vi "系统配置.vi"() -> (3 "线别配置 2":T2={"线别名称"="A157", "LOT NO"="Z-TEST", "机器名"="1", "作业员ID"="A157"})   [LabVIEW 2014]
uses:
  Button.ctl
panel:
  out "线别[]":T1(array[cluster])
  out "作业员IDout":string="A157"
  out "dup path":path caption="路径副本"
  in  "线别设置 2":T3={"LOT NO"="A157", "机器名"="Z-TEST", "QTY"="1", "ACTIVITY"="", "RESOURCE"="A-6-Z-TEST", "NC_CODE"="Z-TEST_FAIL", "IP"="10.9.30.175", "PORT"="50100", "URL"="/manufacturing/IntegrationServlet?InterType=XML&message="}
  out "MES 配置 2":T4={"线别名称"="A157", "LOT NO"="Z-TEST", "机器名"="1"}
  in  "线别配置":T2={"线别名称"="A157", "LOT NO"="Z-TEST", "机器名"="1", "作业员ID"="A157"}
  in  "delete":T5
  in  "input":T5
  in  "新建":T5
  in  "Exit":T5
  in  "所有线别":i32(listbox)
  in  "线别名称":string
  # "用户配置"
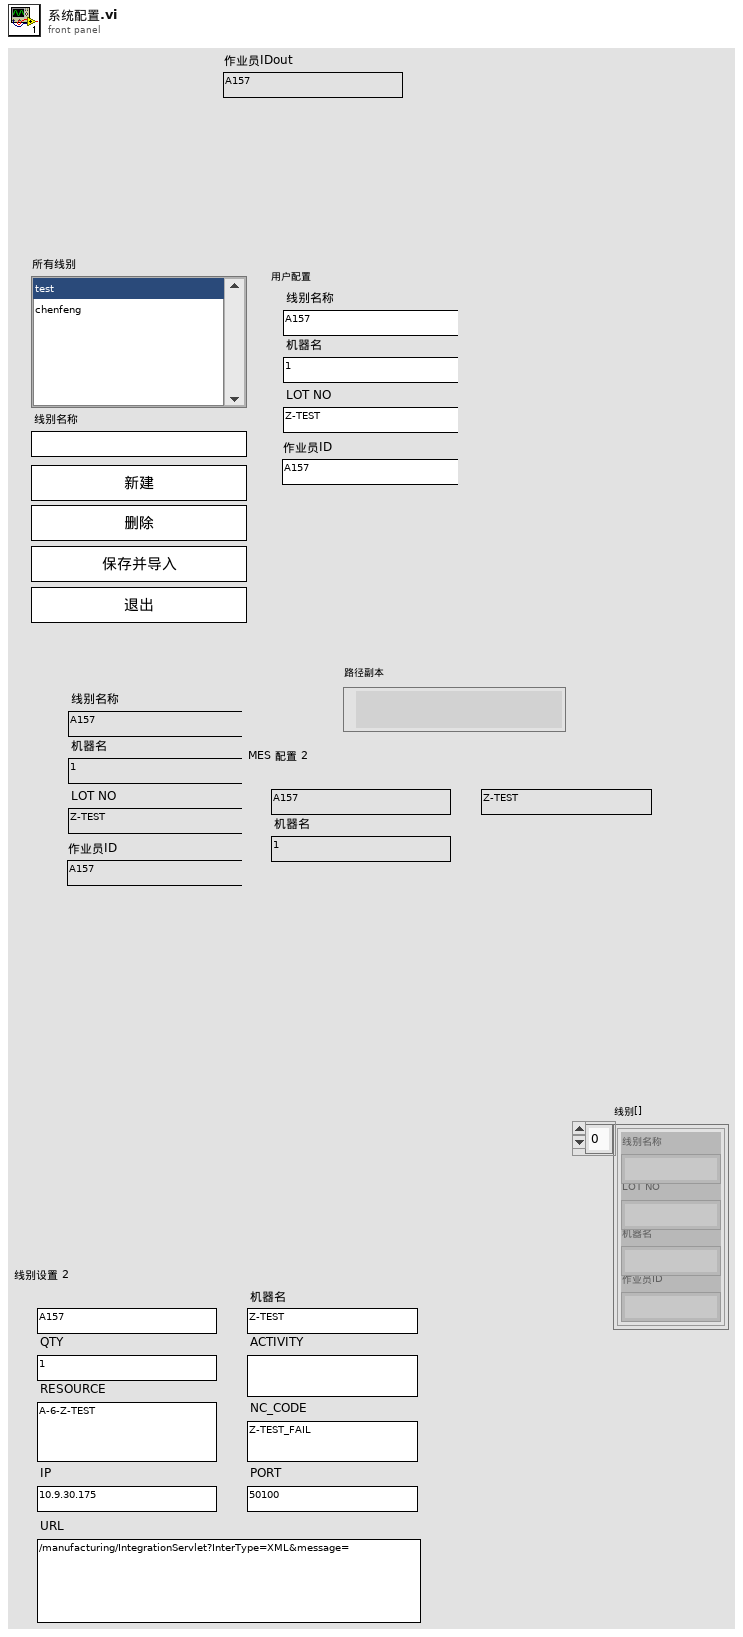
[diagram p1: front panel]
types:
  T1 = cluster{"线别名称":string, "LOT NO":string, "机器名":string, "作业员ID":string}[]
  T2 = cluster{"线别名称":string, "LOT NO":string, "机器名":string, "作业员ID":string}
  T3 = cluster{"LOT NO":string, "机器名":string, "QTY":string, "ACTIVITY":string, "RESOURCE":string, "NC_CODE":string, "IP":string, "PORT":string, "URL":string}
  T4 = cluster{"线别名称":string, "LOT NO":string, "机器名":string}
  T5 = typedef "Button.ctl" = bool
  T6 = cluster{"名称":string, "MES 配置":cluster{"SITE":string, "OPERATION":string, "QTY":string, "ACTIVITY":string, "RESOURCE":string, "NC_CODE":string, "IP":string, "PORT":string, "URL":string}}
  T7 = cluster{"名称":string, "电机位置":cluster{"左工位工作位置":cluster{"Axis":i16, "Distance":i32, "StrVel":i32, "MaxVel":i32}, "左工位抬起开关位置":cluster{"Axis":i16, "Distance":i32, "StrVel":i32, "MaxVel":i32}, "左工位按下开关位置":cluster{"Axis":i16, "Distance":i32, "StrVel":i32, "MaxVel":i32}, "右工位工作位置":cluster{"Axis":i16, "Distance":i32, "StrVel":i32, "MaxVel":i32}, "右工位抬起开关位置":cluster{"Axis":i16, "Distance":i32, "StrVel":i32, "MaxVel":i32}, "右工位按下开关位置":cluster{"Axis":i16, "Distance":i32, "StrVel":i32, "MaxVel":i32}}}
  T8 = cluster{"名称":string, "判定条件":cluster{"A1-A2电阻":cluster{"上限":dbl, "下限":dbl, "单位":string}, "A3-A4电阻":cluster{"上限":dbl, "下限":dbl, "单位":string}, "A4-A5电阻":cluster{"上限":dbl, "下限":dbl, "单位":string}, "A5-A6电阻":cluster{"上限":dbl, "下限":dbl, "单位":string}, "A1-A3电阻":cluster{"上限":dbl, "下限":dbl, "单位":string}, "A2-A6电阻":cluster{"上限":dbl, "下限":dbl, "单位":string}, "A1导地A3-A5电压":cluster{"上限":dbl, "下限":dbl, "单位":string}, "A2导地A6-A5电压":cluster{"上限":dbl, "下限":dbl, "单位":string}, "抬起开关A3-A5电压":cluster{"上限":dbl, "下限":dbl, "单位":string}, "按下开关A6-A5电压":cluster{"上限":dbl, "下限":dbl, "单位":string}, "背光电流":cluster{"上限":dbl, "下限":dbl, "单位":string}, "A1导地A6-A5电压":cluster{"上限":dbl, "下限":dbl, "单位":string}, "A2导地A3-A5电压":cluster{"上限":dbl, "下限":dbl, "单位":string}}}
  T9 = enum16{"open", "replace", "create", "open or create", "replace or create", "replace or create with confirmation"}
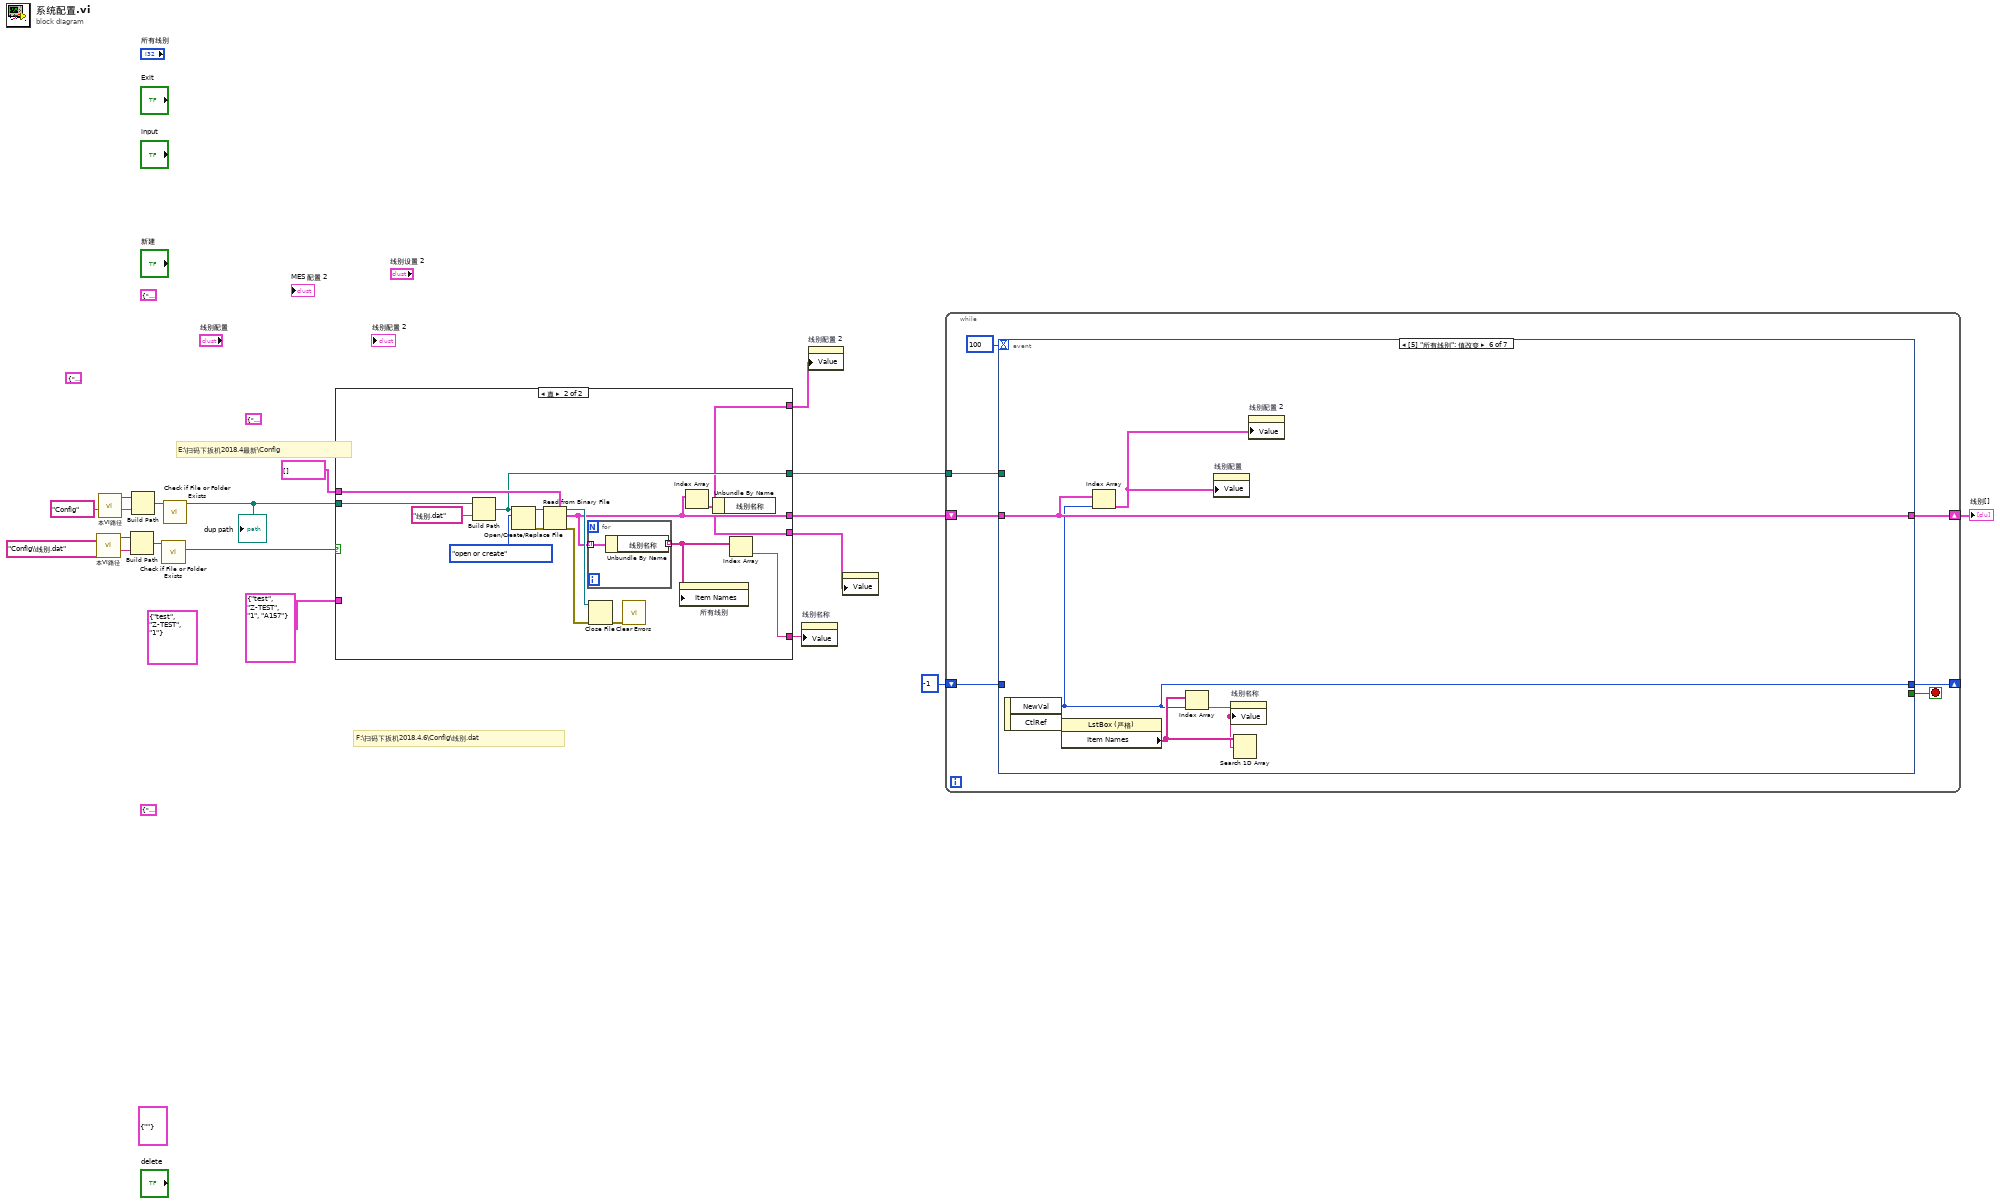
[diagram p0: block diagram]
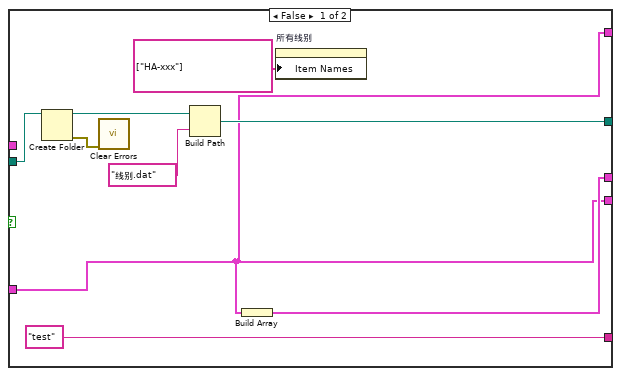
[diagram p2: hidden frame]
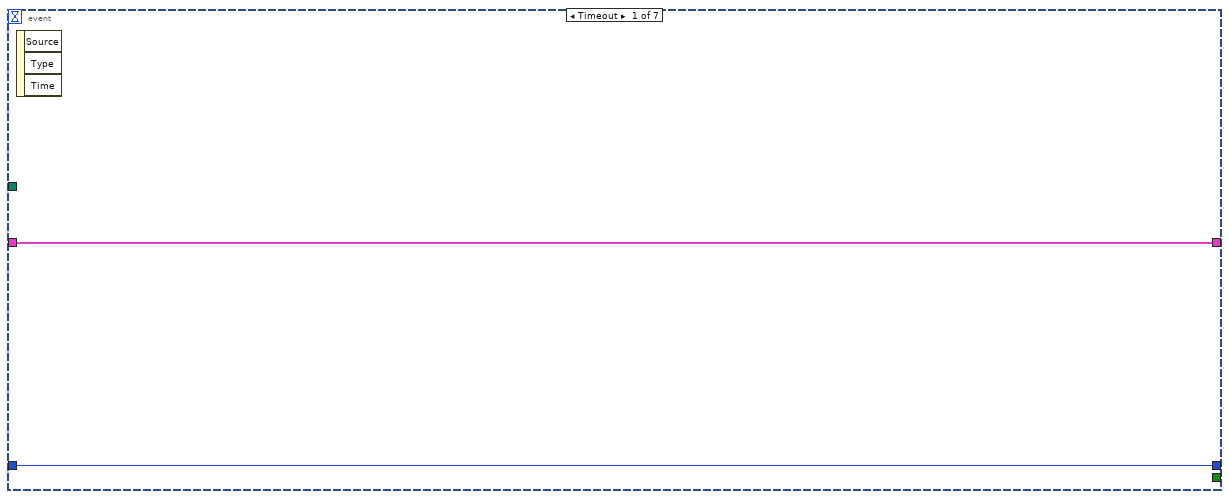
[diagram p3: hidden frame]
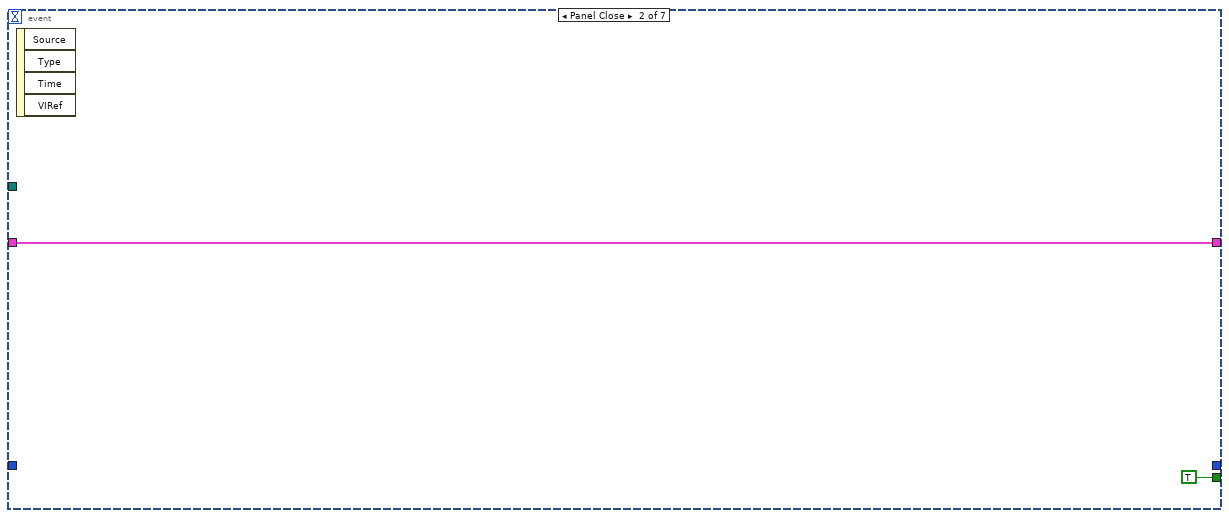
[diagram p4: hidden frame]
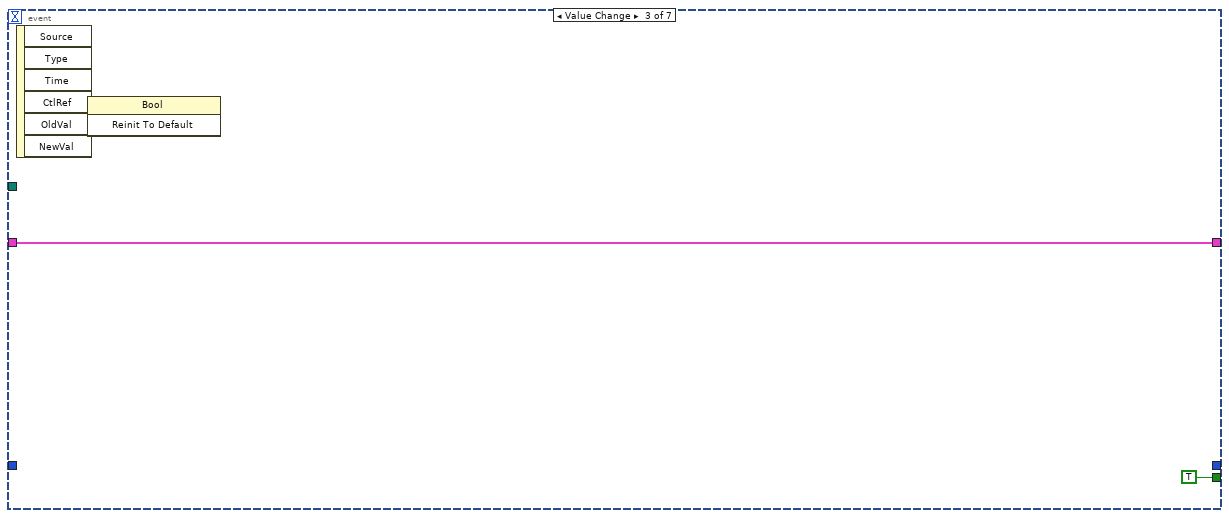
[diagram p5: hidden frame]
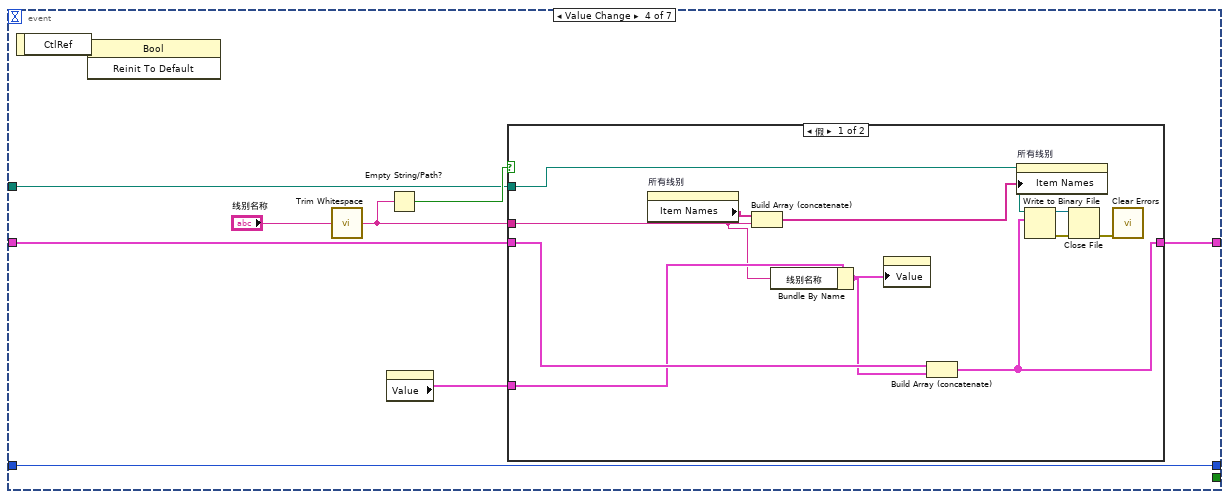
[diagram p6: hidden frame]
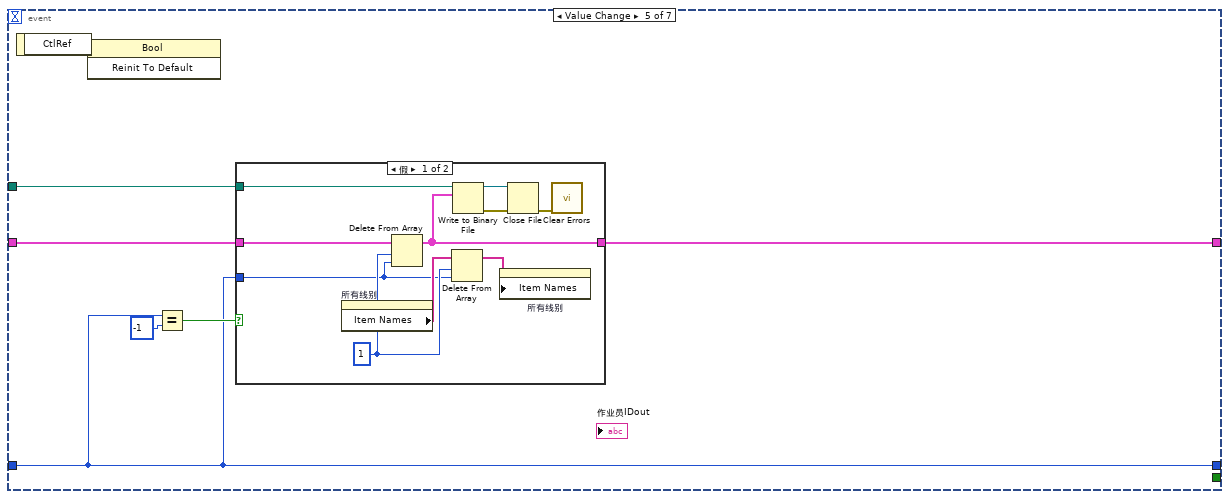
[diagram p8: hidden frame]
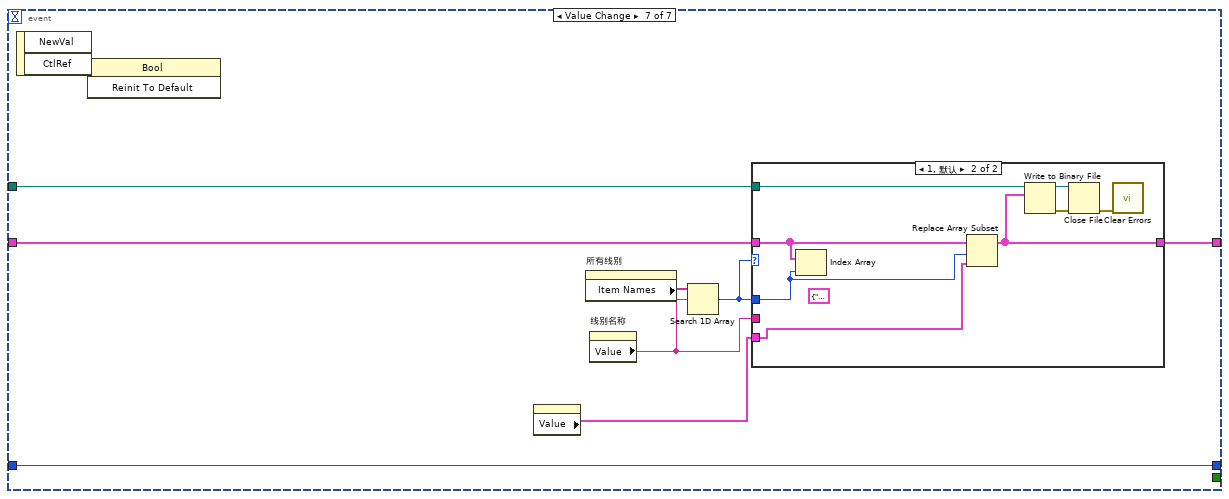
[diagram p10: hidden frame]
diagram:
  (unwired) T4 {"线别名称"="A157", "LOT NO"="Z-TEST", "机器名"="1"} ("线别设置")
  (unwired) T4 {"线别名称"="test", "LOT NO"="Z-TEST", "机器名"="1"} ("线别设置")
  (unwired) T6 {"名称"="Config", "MES 配置"={"SITE"="A157", "OPERATION"="Z-TEST", "QTY"="1", "ACTIVITY"="", "RESOURCE"="A-6-Z-TEST", "NC_CODE"="Z-TEST_FAIL", "IP"="10.9.30.175", "PORT"="50100", "URL"="/manufacturing/IntegrationServlet?InterType=XML&message="}}
  (unwired) T7 {"名称"="Config", "电机位置"={"左工位工作位置"={"Axis"=0, "Distance"=200, "StrVel"=500, "MaxVel"=3000}, "左工位抬起开关位置"={"Axis"=0, "Distance"=200, "StrVel"=500, "MaxVel"=3000}, "左工位按下开关位置"={"Axis"=0, "Distance"=200, "StrVel"=500, "MaxVel"=3000}, "右工位工作位置"={"Axis"=0, "Distance"=200, "StrVel"=500, "MaxVel"=3000}, "右工位抬起开关位置"={"Axis"=0, "Distance"=200, "StrVel"=500, "MaxVel"=3000}, "右工位按下开关位置"={"Axis"=0, "Distance"=200, "StrVel"=500, "MaxVel"=3000}}}
  (unwired) T8 {"名称"="", "判定条件"={"A1-A2电阻"={"上限"=390.0, "下限"=355.0, "单位"="Ω"}, "A3-A4电阻"={"上限"=-1.0, "下限"=-1.0, "单位"=""}, "A4-A5电阻"={"上限"=-1.0, "下限"=-1.0, "单位"="Ω"}, "A5-A6电阻"={"上限"=-1.0, "下限"=-1.0, "单位"="Ω"}, "A1-A3电阻"={"上限"=-1.0, "下限"=-1.0, "单位"="Ω"}, "A2-A6电阻"={"上限"=-1.0, "下限"=-1.0, "单位"="Ω"}, "A1导地A3-A5电压"={"上限"=14.05, "下限"=13.95, "单位"="V"}, "A2导地A6-A5电压"={"上限"=0.0, "下限"=0.0, "单位"="V"}, "抬起开关A3-A5电压"={"上限"=0.0, "下限"=0.0, "单位"="V"}, "按下开关A6-A5电压"={"上限"=0.0, "下限"=0.0, "单位"="V"}, "背光电流"={"上限"=35.0, "下限"=25.0, "单位"="mA"}, "A1导地A6-A5电压"={"上限"=14.05, "下限"=13.95, "单位"="V"}, "A2导地A3-A5电压"={"上限"=0.0, "下限"=0.0, "单位"="V"}}}
  (unwired) cluster{"名称":string} {"名称"=""}
  # "E:\\扫码下扳机2018.4最新\\Config"
  # "F:\\扫码下扳机2018.4.6\\Config\\线别.dat"
  n1 = call "本VI路径.vi"() -> ("stripped path"=w8:path)  [unwired: 11 in]
  n2 = call "本VI路径.vi"() -> ("stripped path"=w10:path)  [unwired: 11 in]
  n3 = Build Path(base path=w8, name or relative path="Config\\线别.dat" ("名称或相对路径")) -> (appended path=w6:path)
  n4 = Build Path(base path=w10, name or relative path="Config" ("名称或相对路径")) -> (appended path=w17:path)
  n5 = call <vilib>:"Check if File or Folder Exists.vi"("path"=w6) -> ("file or folder exists?"=w5:bool)  [unwired: 8 in, 2 out]
  n6 = call <vilib>:"Check if File or Folder Exists.vi"("path"=w17) -> ("dup path"=w15:path)  [unwired: 8 in, 2 out]
  "dup path" <- w15
  n7 = case shown="真" w5 {
    tunnel: w15 -> [w22 w35]
    tunnel: T1 [] -> [_ w38]
    tunnel: T2 {"线别名称"="test", "LOT NO"="Z-TEST", "机器名"="1", "作业员ID"="A157"} ("线别配置") -> [w18 _]
    tunnel: [w19 w37] -> w13
    tunnel: [w20 w34] -> w12
    tunnel: ["test" w29] -> w9
    tunnel: [w18 w27] -> w4
    tunnel: [w18 w27] -> w2
    frame False {
      n8 = Create Folder(path (use dialog)=w22) -> (created path=w23:path, error out=w25:errorcluster)  [unwired: 2 in, 1 out]
      n9 = call <vilib>:"Clear Errors.vi"("error in (no error)"=w25) -> ()  [unwired: 5 in, 2 out]
      n10 = Build Path(base path=w23, name or relative path="线别.dat" ("名称或相对路径")) -> (appended path=w20:path)
      n11 = Build Array(w18) -> (w19:T1)
      n12 = property on="所有线别" class="LstBox (严格)"("Item Names"=string[] ["HA-xxx"] ("项名")) -> ()  [unwired: 2 in, 2 out]
    }
    frame True {
      n13 = Build Path(base path=w35, name or relative path="线别.dat" ("名称或相对路径")) -> (appended path=w34:path)
      n14 = Open/Create/Replace File(file path (use dialog)=w34, operation (0:open)=T9."open or create" ("操作(0:open)")) -> (refnum out=w32:refnum<file>, error out=w28:errorcluster)  [unwired: 4 in, 1 out]
      n15 = Read from Binary File(5:w38, 8:w28, 11:w32) -> (0:w39:errorcluster, 2:w37:T1, 3:w40:refnum<file>)  [unwired: 3 in, 1 out]
      n16 = for {
        tunnel: w37 -> [w42] mode=indexing
        tunnel: [w41] -> w30 mode=indexing
        n17 = Unbundle By Name(w42) -> ("线别名称"=w41:string)
      }
      n18 = Close File(refnum=w40, error in=w39) -> (error out=w36:errorcluster)  [unwired: 1 out]
      n19 = call <vilib>:"Clear Errors.vi"("error in (no error)"=w36) -> ()  [unwired: 5 in, 2 out]
      n20 = property on="所有线别" class="LstBox (严格)"("Item Names"=w30) -> ()  [unwired: 2 in, 2 out]
      n21 = Index Array(array=w37) -> (element=w27:T2)  [unwired: 1 in]
      n22 = Unbundle By Name(w27) -> ()  [unwired: 1 out]
      n23 = Index Array(array=w30) -> (element=w29:string)  [unwired: 1 in]
    }
  }
  n24 = property on="线别名称" class="Str"("Value"=w9) -> ()  [unwired: 2 in, 2 out]
  n25 = property on="线别配置 2" class="Clust (严格)"("Value"=w2) -> ()  [unwired: 2 in, 2 out]
  n26 = property on="线别配置" class="Clust (严格)"("Value"=w4) -> ()  [unwired: 2 in, 2 out]
  n27 = while {
    tunnel: w12 -> [w46]
    shift-right: [w45] -> w1
    shift-left: w13 -> [w47]
    shift-right: [w44] -> _
    shift-left: -1 ("NewVal") -> [w43]
    stop <- w48 stop-if-true
    n28 = event shown="[5] \"所有线别\": 值改变" {
      selector: _ -> [_ _ _ _ _ _ _]
      dyn-events: _ -> [_ _ _ _ _ _ _]
      timeout: 100 -> [_ _ _ _ _ _ _]
      tunnel: [_ TRUE TRUE _ _ _ _] -> w48
      tunnel: w47 -> [w51 w53 w54 w61 w83 w99 w107]
      tunnel: w46 -> [_ _ _ w60 w82 _ w103]
      tunnel: [w51 w53 w54 w59 w81 w99 w105] -> w45
      tunnel: [w50 _ _ w58 w78 w98 w110] -> w44
      tunnel: w43 -> [w50 _ _ w58 w78 _ w110]
      event Timeout {
        n29 = event-data() -> ()  [unwired: 1 in, 3 out]
      }
      event Panel Close {
        n30 = event-data() -> ()  [unwired: 1 in, 4 out]
      }
      event Value Change {
        n31 = event-data() -> ("CtlRef"=w55:refnum<vi>)  [unwired: 1 in, 5 out]
        n32 = invoke class="Bool" method="Reinit To Default"(reference=w55) -> ()  [unwired: 2 in, 3 out]
      }
      event Value Change {
        n33 = event-data() -> ("CtlRef"=w65:refnum<vi>)  [unwired: 1 in]
        n34 = invoke class="Bool" method="Reinit To Default"(reference=w65) -> ()  [unwired: 2 in, 3 out]
        n35 = call <vilib>:"Trim Whitespace.vi"("string"="线别名称") -> ("trimmed string"=w62:string)  [unwired: 1 in]
        n36 = property on="线别配置" class="Clust (严格)"() -> ("Value"=w57:T2)  [unwired: 2 in, 2 out]
        n37 = Empty String/Path?(string/path=w62) -> (empty?=w63:bool)
        n38 = case shown="假" w63 {
          tunnel: w62 -> [w68 _]
          tunnel: w61 -> [w71 w77]
          tunnel: w57 -> [w69 _]
          tunnel: w60 -> [w75 _]
          tunnel: [w70 w77] -> w59
          frame False {
            n39 = property on="所有线别" class="LstBox (严格)"() -> ("Item Names"=w76:string[])  [unwired: 2 in, 2 out]
            n40 = Build Array (concatenate)(w76, w68) -> (w67:string[])
            n41 = Bundle By Name(cluster=w69, "线别名称"=w68) -> (w66:T2)
            n42 = property on="线别配置" class="Clust (严格)"("Value"=w66) -> ()  [unwired: 2 in, 2 out]
            n43 = Build Array (concatenate)(w71, w66) -> (w70:T1)
            n44 = property on="所有线别" class="LstBox (严格)"("Item Names"=w67) -> ()  [unwired: 2 in, 2 out]
            n45 = Write to Binary File(file (use dialog)=w75, data=w70) -> (refnum out=w74:refnum<file>, error out=w73:errorcluster)  [unwired: 4 in, 1 out]
            n46 = Close File(refnum=w74, error in=w73) -> (error out=w72:errorcluster)  [unwired: 1 out]
            n47 = call <vilib>:"Clear Errors.vi"("error in (no error)"=w72) -> ()  [unwired: 5 in, 2 out]
          }
          frame True {
          }
        }
      }
      event Value Change {
        n48 = event-data() -> ("CtlRef"=w84:refnum<vi>)  [unwired: 1 in]
        n49 = invoke class="Bool" method="Reinit To Default"(reference=w84) -> ()  [unwired: 2 in, 3 out]
        n50 = Equal?(x=w78, y=-1) -> (x = y?=w80:bool)
        n51 = case shown="假" w80 {
          tunnel: w83 -> [w88 w95]
          tunnel: w82 -> [w94 _]
          tunnel: [w86 w95] -> w81
          tunnel: w78 -> [w87 _]
          frame False {
            w89 = 1 ("长度")
            n52 = property on="所有线别" class="LstBox (严格)"() -> ("Item Names"=w90:string[])  [unwired: 2 in, 2 out]
            n53 = Delete From Array(array=w88, length=w89, index=w87) -> (array with subset deleted=w86:T1)  [unwired: 1 out]
            n54 = Delete From Array(array=w90, length=w89, index=w87) -> (array with subset deleted=w85:string[])  [unwired: 1 out]
            n55 = Write to Binary File(file (use dialog)=w94, data=w86) -> (refnum out=w93:refnum<file>, error out=w92:errorcluster)  [unwired: 4 in, 1 out]
            n56 = property on="所有线别" class="LstBox (严格)"("Item Names"=w85) -> ()  [unwired: 2 in, 2 out]
            n57 = Close File(refnum=w93, error in=w92) -> (error out=w91:errorcluster)  [unwired: 1 out]
            n58 = call <vilib>:"Clear Errors.vi"("error in (no error)"=w91) -> ()  [unwired: 5 in, 2 out]
          }
          frame True {
          }
        }
      }
      event "所有线别": Value Change {
        n59 = event-data() -> ("NewVal"=w98:i32, "CtlRef"=w101:refnum<vi>)  [unwired: 1 in]
        n60 = property class="LstBox (严格)"(reference=w101) -> ("Item Names"=w100:string[])  [unwired: 1 in, 2 out]
        n61 = Index Array(array=w99, index=w98) -> (element=w96:T2)
        n62 = Index Array(array=w100, index=w98) -> (element=w97:string)
        n63 = property on="线别配置" class="Clust (严格)"("Value"=w96) -> ()  [unwired: 2 in, 2 out]
        n64 = property on="线别名称" class="Str"("Value"=w97) -> ()  [unwired: 2 in, 2 out]
        n65 = Search 1D Array(1D array=w100, element=w97) -> ()  [unwired: 1 in, 1 out]
        n66 = property on="线别配置 2" class="Clust (严格)"("Value"=w96) -> ()  [unwired: 2 in, 2 out]
      }
      event Value Change {
        n67 = event-data() -> ("CtlRef"=w109:refnum<vi>)  [unwired: 1 in, 1 out]
        n68 = invoke class="Bool" method="Reinit To Default"(reference=w109) -> ()  [unwired: 2 in, 3 out]
        n69 = property on="线别配置" class="Clust (严格)"() -> ("Value"=w102:T2)  [unwired: 2 in, 2 out]
        n70 = property on="所有线别" class="LstBox (严格)"() -> ("Item Names"=w108:string[])  [unwired: 2 in, 2 out]
        n71 = property on="线别名称" class="Str"() -> ("Value"=w104:string)  [unwired: 2 in, 2 out]
        n72 = Search 1D Array(1D array=w108, element=w104) -> (index of element=w106:i32)  [unwired: 1 in]
        n73 = case shown="1, 默认" w106 {
          tunnel: w107 -> [w111 w119]
          tunnel: w106 -> [_ w118]
          tunnel: [w111 w114] -> w105
          tunnel: w102 -> [_ w112]
          tunnel: w104 -> [_ _]
          tunnel: w103 -> [_ w113]
          frame -1 {
          }
          frame 1, Default {
            (unwired) T6 {"名称"="Config", "MES 配置"={"SITE"="A157", "OPERATION"="Z-TEST", "QTY"="1", "ACTIVITY"="", "RESOURCE"="A-6-Z-TEST", "NC_CODE"="Z-TEST_FAIL", "IP"="10.9.30.175", "PORT"="50100", "URL"="/manufacturing/IntegrationServlet?InterType=XML&message="}}
            n74 = Index Array(array=w119, index=w118) -> ()  [unwired: 1 out]
            n75 = Replace Array Subset(array=w119, new element=w112, index=w118) -> (w114:T1)
            n76 = Write to Binary File(file (use dialog)=w113, data=w114) -> (refnum out=w117:refnum<file>, error out=w116:errorcluster)  [unwired: 4 in, 1 out]
            n77 = Close File(refnum=w117, error in=w116) -> (error out=w115:errorcluster)  [unwired: 1 out]
            n78 = call <vilib>:"Clear Errors.vi"("error in (no error)"=w115) -> ()  [unwired: 5 in, 2 out]
          }
        }
      }
    }
  }
  "线别[]" <- w1
